vi "Configure Arbitrary Waveform Phase.vi"(6 "Phase Unit (0: Radian)":u16(ring) items=["Radians", "Degrees"], 7 "Phase Level (-1)":dbl=-1.0, 8 "error in (no error)":errorcluster, 10 "Channel (0: Channel 1)":u16(ring) items=["Channel 1", "Channel 2"], 11 "VISA resource name":refnum<visa-resource-name>) -> (0 "error out":errorcluster, 3 "VISA resource name out":refnum<visa-resource-name>)   [LabVIEW 2019, in "Tektronix AFG 3000 Series.lvlib"]
doc: "Configures the phase for arbitrary waveform. Please select the arbitrary waveform and set other values through Configure Arbitrary Waveform.vi."
uses:
  Tektronix AFG 3000 Series.lvlib
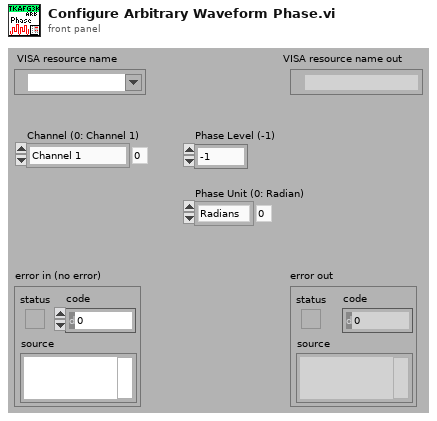
[diagram p1: front panel]
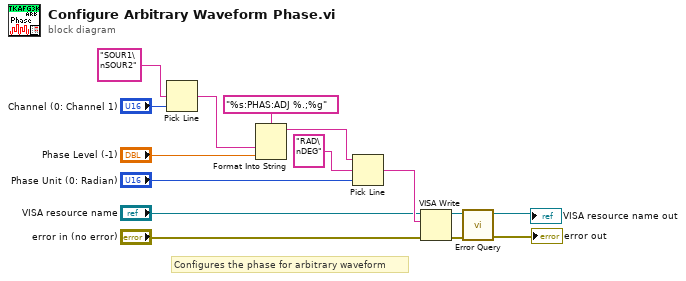
[diagram p0: block diagram]
diagram:
  # "Configures the phase for arbitrary waveform"
  n1 = Pick Line(multi-line string="SOUR1\nSOUR2" ("string (\"\")"), line index="Channel (0: Channel 1)") -> (output string=w1:string)  [unwired: 1 in]
  n2 = Format Into String(format string="%s:PHAS:ADJ %.;%g", w1, "Phase Level (-1)") -> (resulting string=w13:string)  [unwired: 2 in, 1 out]
  n3 = Pick Line(string ("")=w13, multi-line string="RAD\nDEG", line index="Phase Unit (0: Radian)") -> (output string=w6:string)
  n4 = VISA Write(VISA resource name="VISA resource name", write buffer=w6, error in (no error)="error in (no error)") -> (VISA resource name out=w8:refnum<visa-resource-name>, error out=w7:errorcluster)  [unwired: 1 out]
  n5 = call "Error Query.vi"("error in (no error)"=w7, "VISA resource name"=w8) -> ("error out"=→"error out":errorcluster, "VISA resource name out"=→"VISA resource name out":refnum<visa-resource-name>)  [unwired: 6 in, 2 out]
